vi "ReadCount.vi"(11 "TypedCircularBuffer in":refnum<class "VarCircularBuffer.lvclass">) -> (2 "Count":u32, 3 "TypedCircularBuffer out":refnum<class "VarCircularBuffer.lvclass">)   [LabVIEW 2024, in "VarCircularBuffer.lvclass"]
uses:
  VarCircularBuffer.lvclass
  VarCircularBuffer.lvclass/VarCircularBuffer.ctl
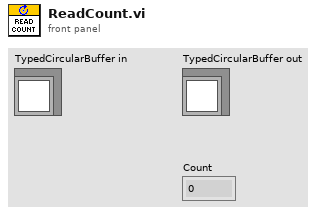
[diagram p1: front panel]
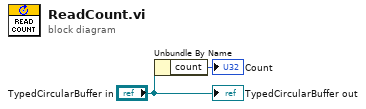
[diagram p0: block diagram]
diagram:
  n1 = Unbundle By Name("TypedCircularBuffer in") -> ("count"=→"Count":u32)
  "TypedCircularBuffer out" <- "TypedCircularBuffer in"
